vi "RSZVB Get Calibration Data Timestamp.vi"(8 "error in (no error)":errorcluster {"code" format="%.0x"}, 9 "Calibration (1)":i32=1, 10 "Channel (1)":i32=1, 11 "VISA session":refnum<visa-resource-name>) -> (0 "error out":errorcluster {"code" format="%.0x"}, 2 "Timestamp":string, 3 "dup VISA session":refnum<visa-resource-name>)   [LabVIEW 2011]
doc: "This VI queries the timestamp of the calibration in 24-hour clock.\n\nRemote-control command(s):\n[SENSe<Ch>:]CORRection:DATA:PARameter<Cal>? TSTamp"
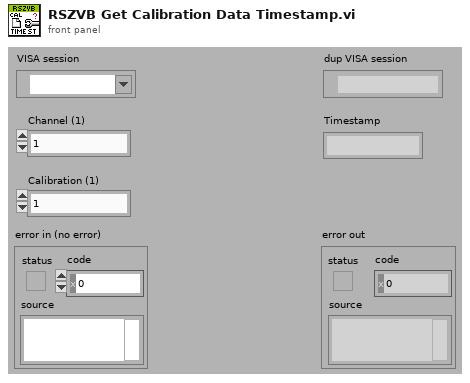
[diagram p1: front panel]
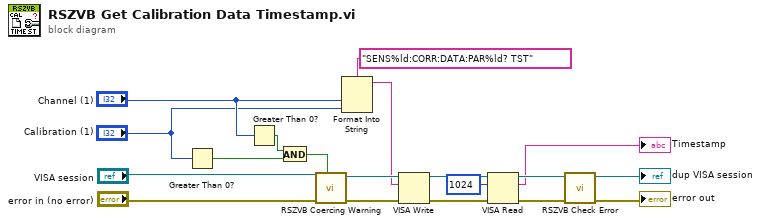
[diagram p0: block diagram]
diagram:
  n1 = Greater Than 0?(x="Calibration (1)") -> (x > 0?=w3:bool)
  n2 = Greater Than 0?(x="Channel (1)") -> (x > 0?=w4:bool)
  n3 = And(x=w4, y=w3) -> (x .and. y?=w5:bool)
  n4 = call "RSZVB Coercing Warning.vi"("In Range?"=w5, "error in (no error)"="error in (no error)", "VISA session"="VISA session") -> ("error out"=w13:errorcluster, "dup VISA session"=w14:refnum<visa-resource-name>)  [unwired: 7 in]
  n5 = Format Into String(format string="SENS%ld:CORR:DATA:PAR%ld? TST", "Channel (1)", "Calibration (1)") -> (resulting string=w11:string)  [unwired: 2 in, 1 out]
  n6 = VISA Write(VISA resource name=w14, write buffer=w11, error in (no error)=w13) -> (VISA resource name out=w18:refnum<visa-resource-name>, error out=w19:errorcluster)  [unwired: 1 out]
  n7 = VISA Read(VISA resource name=w18, byte count=u32 1024, error in (no error)=w19) -> (VISA resource name out=w15:refnum<visa-resource-name>, read buffer=→"Timestamp":string, error out=w16:errorcluster)  [unwired: 1 out]
  n8 = call "RSZVB Check Error.vi"("error in (no error)"=w16, "VISA session"=w15) -> ("error out"=→"error out":errorcluster, "dup VISA session"=→"dup VISA session":refnum<visa-resource-name>)  [unwired: 8 in]
